vi "read.vi"(8 "error in":errorcluster, 9 "timeout in ms (-1)":i32=-1, 11 "identifying queue in":refnum<class "identifying queue.lvclass">) -> (0 "error out":errorcluster, 1 "timed out?":bool, 2 "message":refnum<class "communicator message.lvclass">)   [LabVIEW 2015, in "identifying queue.lvclass"]
uses:
  identifying queue.lvclass
  message/communicator message.lvclass
  identifying queue.lvclass/identifying queue.ctl
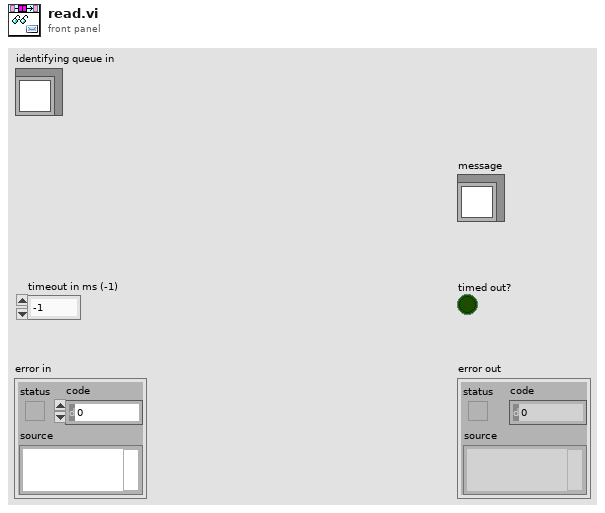
[diagram p1: front panel]
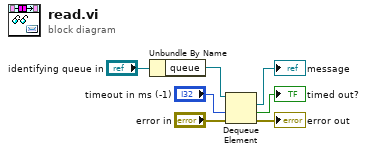
[diagram p0: block diagram]
diagram:
  n1 = Unbundle By Name("identifying queue in") -> ("queue"=w4:refnum<queue>)
  n2 = Dequeue Element(queue=w4, timeout in ms (-1)="timeout in ms (-1)", error in (no error)="error in") -> (element=→"message":refnum<class "communicator message.lvclass">, timed out?=→"timed out?":bool, error out=→"error out":errorcluster)  [unwired: 1 out]
